vi "Call.vi"(7 "Cache Ref (F)":bool, 8 "error in (no error)":errorcluster, 9 "Inputs":variant, 10 "Method Name":string, 11 "SMOFacade in":refnum<class "SMOFacade.lvclass">) -> (0 "error out":errorcluster, 1 "Outputs":variant, 2 "Method Name dup":string, 3 "SMOFacade out":refnum<class "SMOFacade.lvclass">)   [LabVIEW 2013, in "SMOFacade.lvclass"]
uses:
  SMOFacade.lvclass
  Registry/SMO_API--Cluster.ctl
  Terminal/SMOTerminal.lvclass
  SMOFacade.lvclass/SMOFacade.ctl
  Registry/Registry-SMO.lvclass
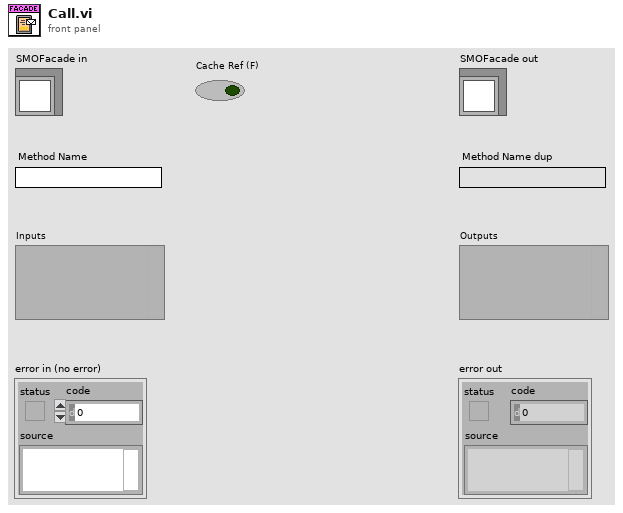
[diagram p1: front panel]
types:
  T1 = typedef "Registry-SMO.lvclass/SMO_API--Cluster.ctl" = cluster{"Method Name":string, "Full Method Name":string, "SMO Input":refnum<class "SMOTerminal.lvclass">, "SMO Output":refnum<class "SMOTerminal.lvclass">, "Inputs":refnum<class "SMOTerminal.lvclass">[], "Outputs":refnum<class "SMOTerminal.lvclass">[], "Error Output":refnum<class "SMOTerminal.lvclass">, "vi reference":refnum<vi>}
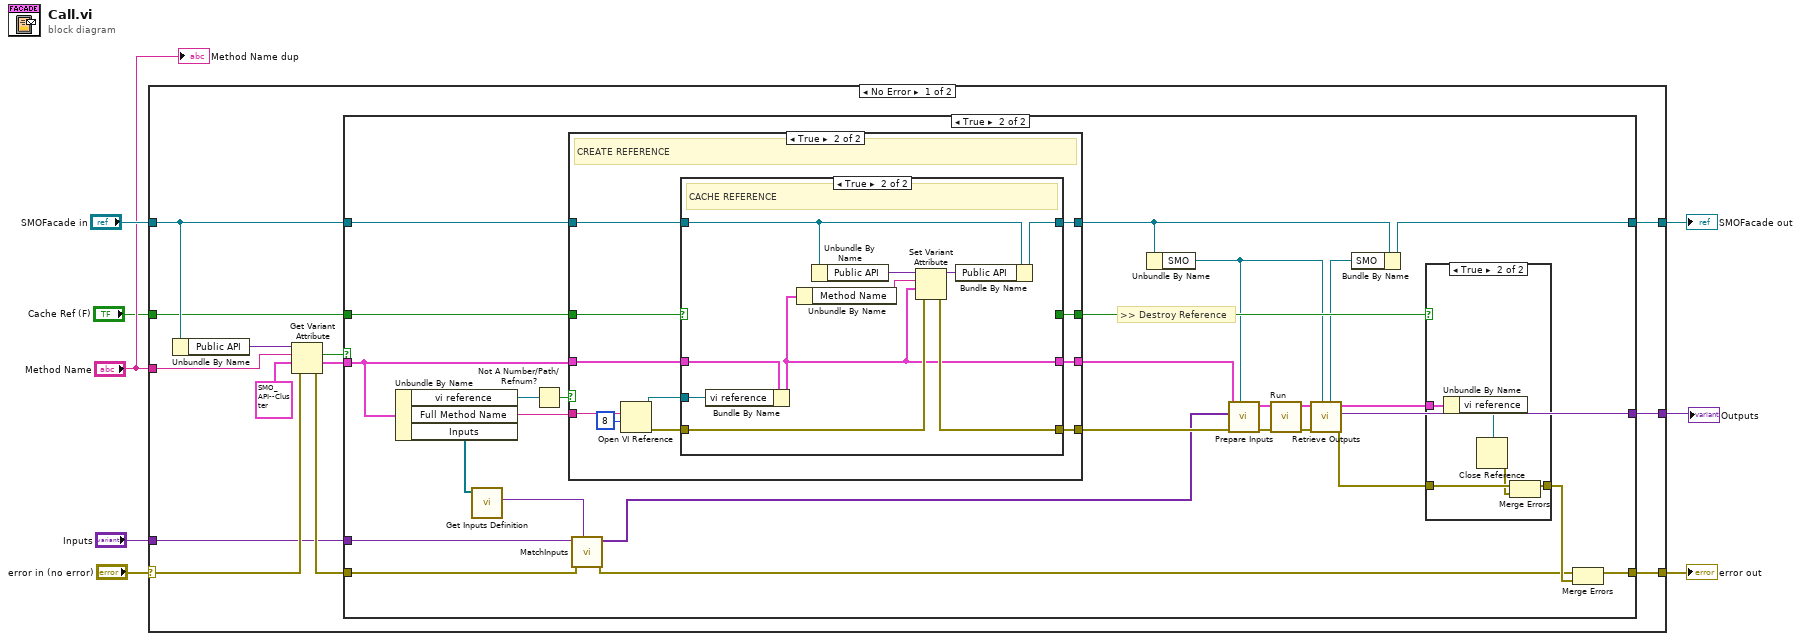
[diagram p0: block diagram]
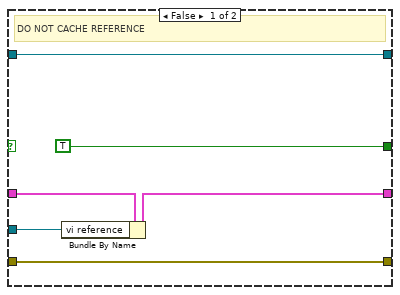
[diagram p5: hidden frame]
diagram:
  n1 = case shown="No Error" "error in (no error)" {
    selector: "error in (no error)" -> [w18 w90]
    tunnel: "SMOFacade in" -> [w21 w91]
    tunnel: [w16 w91] -> w7
    tunnel: "Method Name" -> [w9 _]
    tunnel: [w14 w90] -> w5
    tunnel: "Inputs" -> [w12 _]
    tunnel: [w11 _] -> w2
    tunnel: "Cache Ref (F)" -> [w10 _]
    frame No Error {
      n2 = Unbundle By Name(w21) -> ("Public API"=w20:variant)
      n3 = Get Variant Attribute(Variant=w20, name=w9, default value (empty Variant)=T1 {"Method Name"="", "Full Method Name"="", "SMO Input"=refnum, "SMO Output"=refnum, "Inputs"=[], "Outputs"=[], "Error Output"=refnum, "vi reference"=refnum} ("API"), error in=w18) -> (found=w17:bool, value=w13:T1, error out=w15:errorcluster)  [unwired: 1 out]
      n4 = case shown="True" w17 {
        tunnel: w21 -> [w26 w47]
        tunnel: [w26 w44] -> w16
        tunnel: w15 -> [w25 w28]
        tunnel: [w24 w39] -> w14
        tunnel: w13 -> [_ w46]
        tunnel: w12 -> [_ w31]
        tunnel: [_ w54] -> w11
        tunnel: w10 -> [_ w48]
        frame False {
          n5 = call <vilib>:"Error Cluster From Error Code.vi"("error in (no error)"=w25, "error message (\"\")"="Method Name not found.", "error code (0)"=1) -> ("error out"=w24:errorcluster)  [unwired: 6 in]
        }
        frame True {
          # ">> Destroy Reference"
          n6 = Unbundle By Name(w46) -> ("vi reference"=w49:refnum<vi>, "Full Method Name"=w53:string, "Inputs"=w32:refnum<class "SMOTerminal.lvclass">[])
          n7 = call "Get Inputs Definition.vi"("Inputs"=w32) -> ("Default Input"=w30:variant)  [unwired: 9 in, 1 out]
          n8 = Not A Number/Path/Refnum?(number/path/refnum=w49) -> (NaN/Path/Refnum?=w50:bool)
          n9 = case shown="True" w50 {
            tunnel: w53 -> [_ w73]
            tunnel: [_ w67] -> w51
            tunnel: w48 -> [_ w65]
            tunnel: w47 -> [w62 w71]
            tunnel: [w62 w70] -> w42
            tunnel: w46 -> [w61 w69]
            tunnel: [w61 w66] -> w41
            tunnel: [_ w63] -> w45
            frame False {
              # "REFERENCE ALREADY CACHED"
            }
            frame True {
              # "CREATE REFERENCE"
              n10 = Open VI Reference(vi path=w73, options=8) -> (vi reference=w64:refnum<vi>, error out=w68:errorcluster)  [unwired: 4 in]
              n11 = case shown="True" w65 {
                tunnel: w71 -> [w79 w89]
                tunnel: [w79 w88] -> w70
                tunnel: w69 -> [w75 w85]
                tunnel: w64 -> [w76 w80]
                tunnel: w68 -> [w78 w84]
                tunnel: [w78 w83] -> w67
                tunnel: [w74 w81] -> w66
                tunnel: [TRUE _] -> w63
                frame False {
                  # "DO NOT CACHE REFERENCE"
                  n12 = Bundle By Name(cluster=w75, "vi reference"=w76) -> (w74:T1)
                }
                frame True {
                  # "CACHE REFERENCE"
                  n13 = Bundle By Name(cluster=w85, "vi reference"=w80) -> (w81:T1)
                  n14 = Unbundle By Name(w81) -> ("Method Name"=w82:string)
                  n15 = Unbundle By Name(w89) -> ("Public API"=w87:variant)
                  n16 = Set Variant Attribute(Variant=w87, name=w82, value=w81, error in=w84) -> (Variant out=w86:variant, error out=w83:errorcluster)  [unwired: 1 out]
                  n17 = Bundle By Name(cluster=w89, "Public API"=w86) -> (w88:refnum<class "SMOFacade.lvclass">)
                }
              }
            }
          }
          n18 = call "MatchInputs.vi"("type to match"=w30, "error in"=w28, "Inputs"=w31) -> ("error out"=w27:errorcluster, "Matched Inputs"=w29:variant[])  [unwired: 6 in, 1 out]
          n19 = Unbundle By Name(w42) -> ("SMO"=w33:refnum<class "SMO.lvclass">)
          n20 = call "Prepare Inputs.vi"("SMO"=w33, "error in (no error)"=w51, "Inputs"=w29, "API"=w41) -> ("error out"=w52:errorcluster, "API dup"=w40:T1)  [unwired: 6 in]
          n21 = call "Run.vi"("error in (no error)"=w52, "API"=w40) -> ("error out"=w43:errorcluster, "API dup"=w35:T1)  [unwired: 8 in]
          n22 = call "Retrieve Outputs.vi"("SMO in"=w33, "error in (no error)"=w43, "API"=w35) -> ("error out"=w37:errorcluster, "Output"=w54:variant, "API dup"=w34:T1, "SMO out"=w36:refnum<class "SMO.lvclass">)  [unwired: 5 in]
          n23 = Bundle By Name(cluster=w42, "SMO"=w36) -> (w44:refnum<class "SMOFacade.lvclass">)
          n24 = case shown="True" w45 {
            tunnel: w37 -> [w55 w58]
            tunnel: [w55 w56] -> w38
            tunnel: w34 -> [_ w59]
            frame False {
            }
            frame True {
              n25 = Unbundle By Name(w59) -> ("vi reference"=w60:refnum<vi>)
              n26 = Close Reference(reference=w60) -> (error out=w57:errorcluster)  [unwired: 1 in]
              n27 = Merge Errors(w58, w57) -> (w56:errorcluster)
            }
          }
          n28 = Merge Errors(w27, w38) -> (w39:errorcluster)
        }
      }
    }
    frame Error {
    }
  }
  "error out" <- w5
  "SMOFacade out" <- w7
  "Outputs" <- w2
  "Method Name dup" <- "Method Name"
